vi "Close file.vi"(8 "error in (no error)":errorcluster, 11 "file refs":T1 {"file" format="%.0x"}) -> (0 "error out":errorcluster)   [LabVIEW 2013]
uses:
  File refs.ctl
  <vilib>/addons/h5labview2/base/hid_t.ctl
  <vilib>/addons/h5labview2/dataset/H5D.lvlib
  <vilib>/addons/h5labview2/file/H5F.lvlib
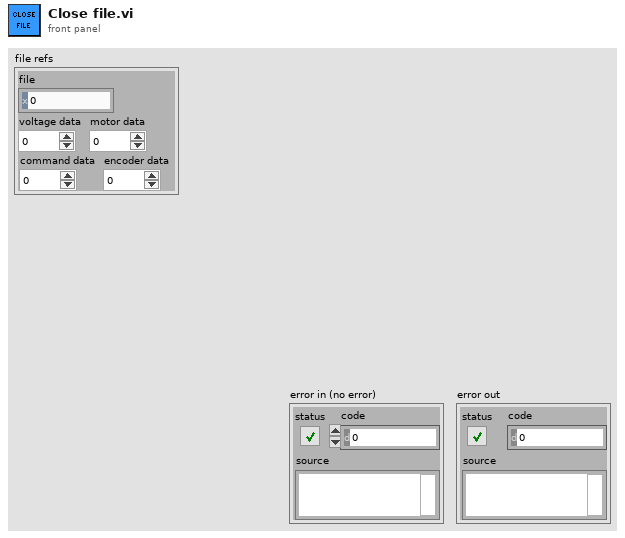
[diagram p1: front panel]
types:
  T1 = typedef "File refs.ctl" = cluster{"file":T2, "voltage data":i32, "motor data":i32, "command data":i32, "encoder data":i32}
  T2 = typedef "hid_t.ctl" = i32
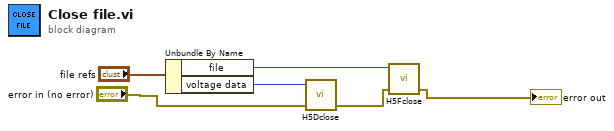
[diagram p0: block diagram]
diagram:
  n1 = Unbundle By Name("file refs") -> ("file"=w2:T2, "voltage data"=w3:i32)
  n2 = call <vilib>:"H5Dclose.vi"("error in (no error)"="error in (no error)", "dset in"=w3) -> ("error out"=w1:errorcluster)  [unwired: 3 in]
  n3 = call <vilib>:"H5Fclose.vi"("error in (no error)"=w1, "ref"=w2) -> ("error out"=→"error out":errorcluster)  [unwired: 3 in]
